vi "Set_Pulse_Single_Channel.vi"(0 "VISA arduino in":refnum<visa-resource-name>, 1 "chanel":u8=2 min=2 max=13 step=1, 2 "Times":dbl[](array[numeric]), 3 "error in":errorcluster, 4 "Check times?":bool) -> (5 "VISA arduino out":refnum<visa-resource-name>, 6 "error out":errorcluster)   [LabVIEW 2021]
uses:
  <vilib>/Utility/error.llb/Error Cluster From Error Code.vi
  <vilib>/ErrorRing/Error Ring.xnode
panel:
  out "delay":u32
  # "Private"
  # "Public"
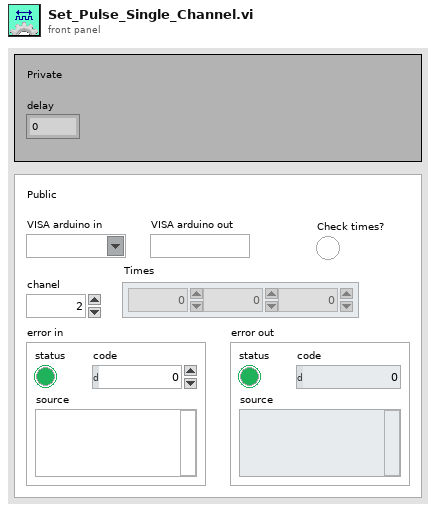
[diagram p1: front panel]
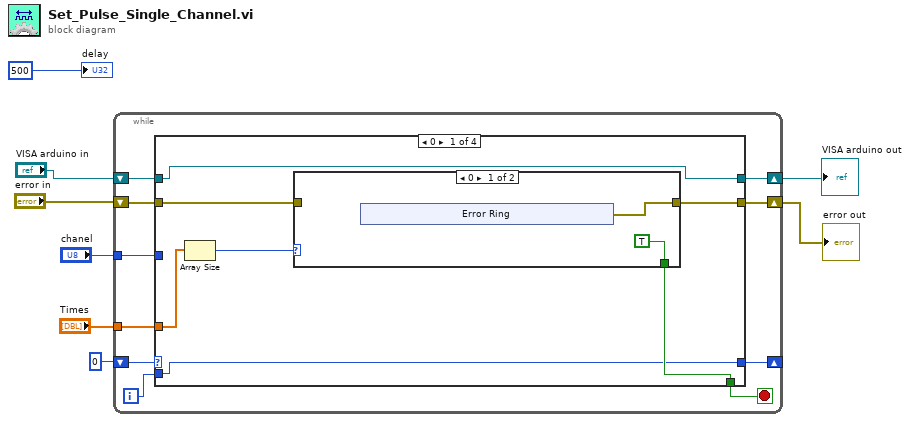
[diagram p0: block diagram]
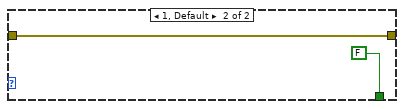
[diagram p2: hidden frame]
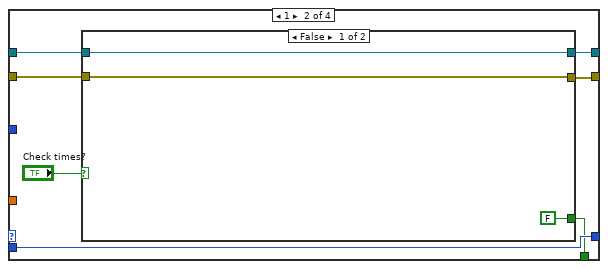
[diagram p3: hidden frame]
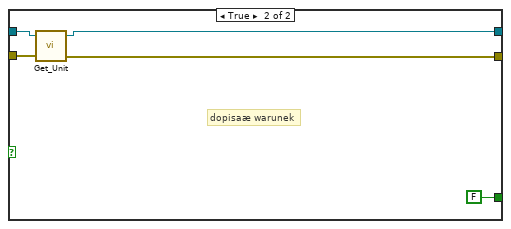
[diagram p4: hidden frame]
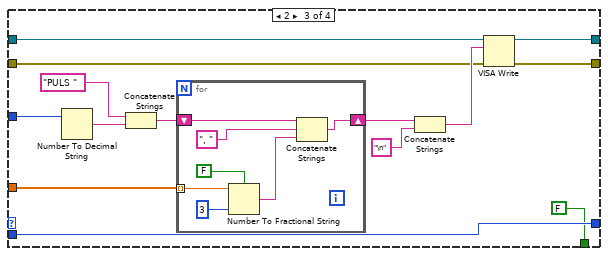
[diagram p5: hidden frame]
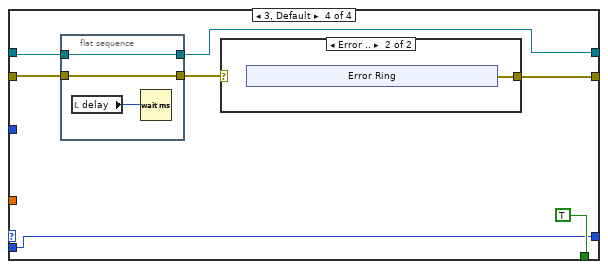
[diagram p6: hidden frame]
diagram:
  n1 = while {
    shift-right: [w10] -> _
    shift-left: 0 -> [w18]
    tunnel: "Times" -> [w16]
    shift-right: [w11] -> w2
    shift-left: "VISA arduino in" -> [w14]
    shift-right: [w13] -> w1
    shift-left: "error in" -> [w15]
    tunnel: "chanel" -> [w9]
    i -> [w17]
    stop <- w12 stop-if-true
    n2 = case shown="0" w18 {
      tunnel: w17 -> [w19 w36 w51 w76]
      tunnel: w16 -> [w25 _ w58 _]
      tunnel: w15 -> [w23 w39 w52 w73]
      tunnel: w14 -> [w20 w40 w53 w71]
      tunnel: [w22 w37 w55 w75] -> w13
      tunnel: [w21 w35 FALSE TRUE] -> w12
      tunnel: [w20 w38 w54 w72] -> w11
      tunnel: [w19 w36 w51 w76] -> w10
      tunnel: w9 -> [_ _ w57 _]
      frame 0 {
        n3 = Array Size(array=w25) -> (size(s)=w24:i32)
        n4 = case shown="0" w24 {
          tunnel: w23 -> [_ w34]
          tunnel: [w27 w34] -> w22
          tunnel: [TRUE FALSE] -> w21
          frame 0 {
            n5 = xnode "Error Ring"() -> ("error out"=w27:errorcluster)
          }
          frame 1, Default {
          }
        }
      }
      frame 1 {
        n6 = case shown="False" "Check times?" {
          tunnel: w40 -> [w44 w49]
          tunnel: w39 -> [w43 w48]
          tunnel: [w44 w47] -> w38
          tunnel: [w43 w46] -> w37
          tunnel: [FALSE FALSE] -> w35
          frame False {
          }
          frame True {
            # "dopisaæ warunek"
            n7 = call "Get_Unit.vi"("error in"=w48, "VISA arduino in"=w49) -> ("error out"=w46:errorcluster, "VISA arduino out"=w47:refnum<visa-resource-name>)  [unwired: 1 in, 1 out]
          }
        }
      }
      frame 2 {
        n8 = Number To Decimal String(number=w57) -> (decimal integer string=w63:string)  [unwired: 1 in]
        n9 = Concatenate Strings("PULS " ("string"), w63) -> (w61:string)
        n10 = for {
          tunnel: w58 -> [w68] mode=indexing
          shift-right: [w70] -> w60
          shift-left: w61 -> [w69]
          n11 = Number To Fractional String(use system decimal point (T)=FALSE, number=w68, precision (6)=i16 3) -> (F-format string=w65:string)  [unwired: 1 in]
          n12 = Concatenate Strings(w69, ", " ("string"), w65) -> (w70:string)
        }
        n13 = Concatenate Strings(w60, "\n" ("string")) -> (w56:string)
        n14 = VISA Write(VISA resource name=w53, write buffer=w56, error in (no error)=w52) -> (VISA resource name out=w54:refnum<visa-resource-name>, error out=w55:errorcluster)  [unwired: 1 out]
      }
      frame 3, Default {
        n15 = flat-sequence {
          tunnel: [w79] -> w74
          tunnel: w73 -> [w79]
          tunnel: [w78] -> w72
          tunnel: w71 -> [w78]
          frame #0 {
            n16 = local read "delay"() -> (w80:u32)
            n17 = Wait (ms)(milliseconds to wait=w80) -> ()  [unwired: 1 out]
          }
        }
        n18 = case shown="Error .." w74 {
          selector: w74 -> [w81 _]
          tunnel: [w81 w82] -> w75
          frame No Error {
          }
          frame Error {
            n19 = xnode "Error Ring"() -> ("error out"=w82:errorcluster)
          }
        }
      }
    }
  }
  "error out" <- w1
  "VISA arduino out" <- w2
  "delay" <- u32 500
